vi "Timing_GCFS.vi"(0 "?":T1 {"Data Out Cluster"."Particle Measurements (Pixels) (Particle Analysis 1)" format="%.2f"}) -> (1 "Sample dt (ms)":i64, 2 "Sample dt (s)":dbl)   [LabVIEW 2024]
uses:
  DataCluster_GCFS.ctl
  <vilib>/userDefined/High Color/IMAQdx.ctl
  <vilib>/vision/Image Controls.llb/IMAQ Image.ctl
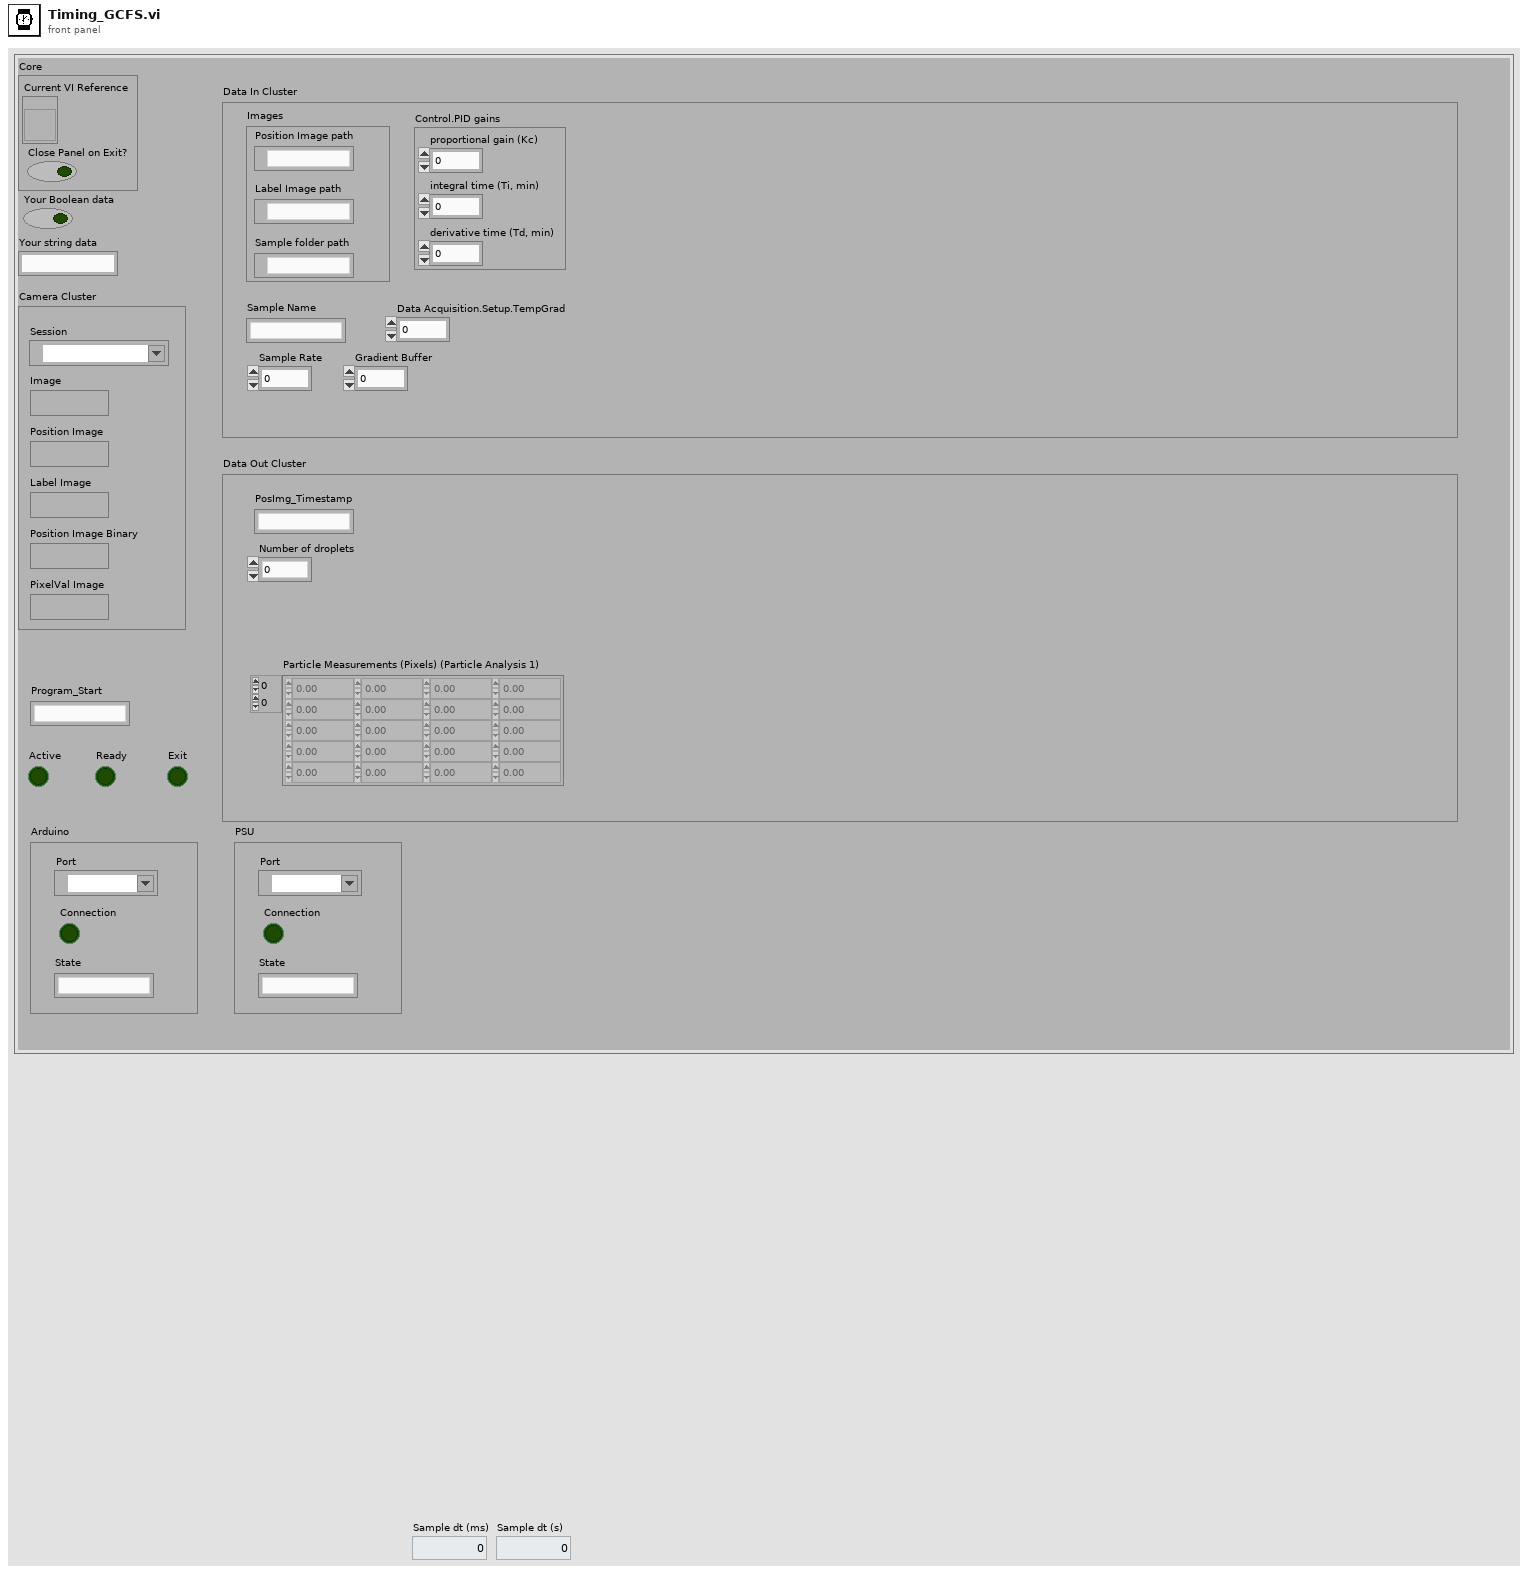
[diagram p1: front panel]
types:
  T1 = typedef "DataCluster_GCFS.ctl" = cluster{"Core":cluster{"Current VI Reference":refnum<vi>, "Close Panel on Exit?":bool}, "Your Boolean data":bool, "Your string data":string, "Camera Cluster":cluster{"Session":T2, "Image":T3, "Position Image":T3, "PixelVal Image":T3, "Position Image Binary":T3, "Lable Image":T3}, "Data In Cluster":cluster{"Images":cluster{"Position Image path":path, "Sample folder path":path, "Label Image path":path}, "Sample Name":string, "Sample Rate":i32, "Gradient Buffer":i32, "Data Acquisition.Setup.TempGrad":dbl, "Control.PID gains":cluster{"proportional gain (Kc)":dbl, "integral time (Ti, min)":dbl, "derivative time (Td, min)":dbl}}, "Active":bool, "Ready":bool, "Exit":bool, "Arduino":cluster{"Connection":bool, "Port":refnum<visa-resource-name>, "State":string}, "Program_Start":string, "Data Out Cluster":cluster{"Particle Measurements (Pixels) (Particle Analysis 1)":dbl[][], "Number of droplets":i32, "PosImg_Timestamp":string}, "PSU":cluster{"Connection":bool, "Port":refnum<visa-resource-name>, "State":string}}
  T2 = typedef "IMAQdx.ctl" = refnum<k21>
  T3 = typedef "IMAQ Image.ctl" = refnum<image>
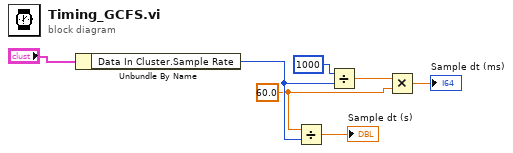
[diagram p0: block diagram]
diagram:
  w3 = 60.0 ("y")
  n1 = Unbundle By Name("?") -> ("Data In Cluster.Sample Rate"=w4:i32)
  n2 = Divide(x=w3, y=w4) -> (x/y=→"Sample dt (s)":dbl)
  n3 = Divide(x=1000, y=w4) -> (x/y=w6:dbl)
  n4 = Multiply(x=w6, y=w3) -> (x*y=→"Sample dt (ms)":dbl)
